vi "Merge Lists.vi"(8 "error in":errorcluster, 9 "new list in":T1[](array[typedef]) {"Last Updated" format="%<%x>T"}, 11 "list in":T1[](array[typedef]) {"Last Updated" format="%<%x>T"}) -> (0 "error out":errorcluster, 3 "list out":T1[](array[typedef]) {"Last Updated" format="%<%x>T"})   [LabVIEW 2018]
uses:
  SR Cluster.ctl
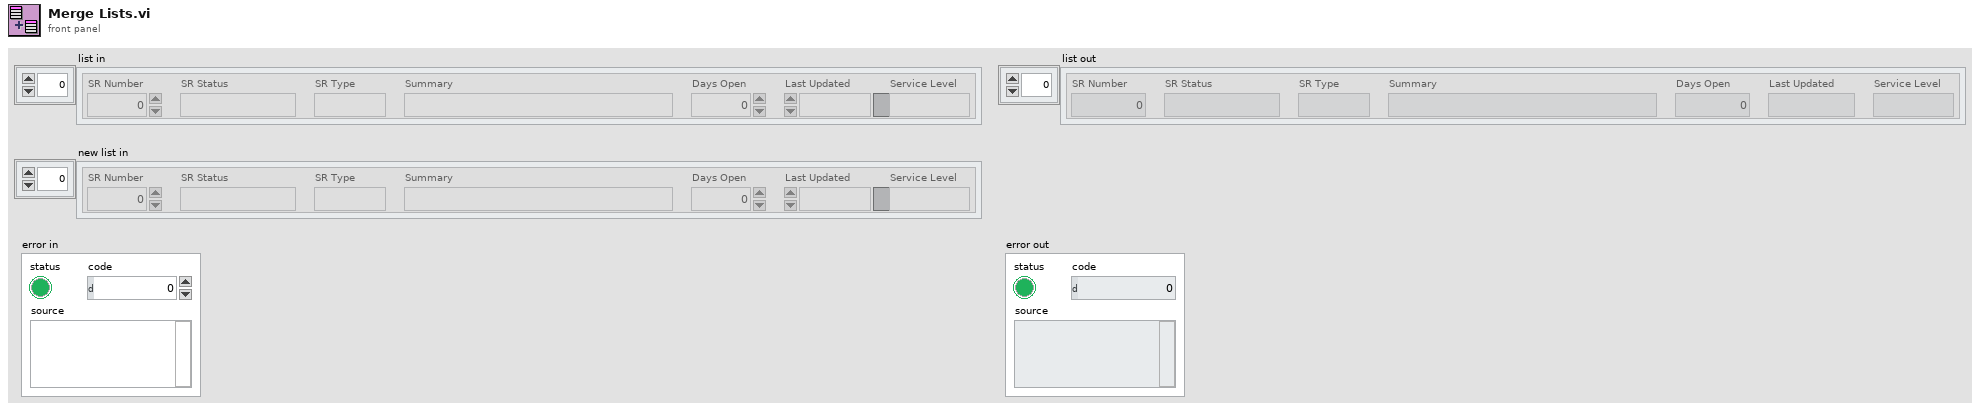
[diagram p1: front panel]
types:
  T1 = typedef "SR Cluster.ctl" = cluster{"SR Number":i32, "SR Status":string, "SR Type":string, "Summary":string, "Days Open":dbl, "Last Updated":timestamp, "Service Level":string}
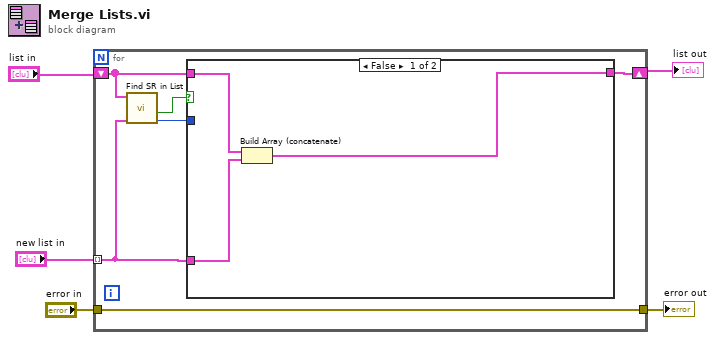
[diagram p0: block diagram]
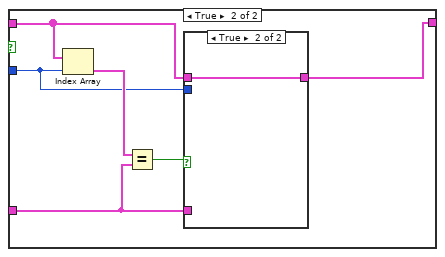
[diagram p2: hidden frame]
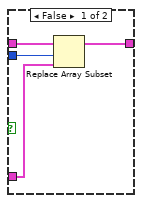
[diagram p3: hidden frame]
diagram:
  n1 = for {
    tunnel: [w11] -> w3
    tunnel: "error in" -> [w11]
    tunnel: "new list in" -> [w8] mode=indexing
    shift-right: [w7] -> w2
    shift-left: "list in" -> [w9]
    n2 = call "Find SR in List.vi"("new SR"=w8, "SR list in"=w9) -> ("SR Index"=w6:i32, "Is SR in List?"=w10:bool)  [unwired: 8 in]
    n3 = case shown="False" w10 {
      tunnel: w9 -> [w14 w18]
      tunnel: w8 -> [w13 w16]
      tunnel: [w12 w15] -> w7
      tunnel: w6 -> [_ w17]
      frame False {
        n4 = Build Array (concatenate)(w14, w13) -> (w12:T1[])
      }
      frame True {
        n5 = Index Array(array=w18, index=w17) -> (element=w19:T1)
        n6 = Equal?(x=w19, y=w16) -> (x = y?=w20:bool)
        n7 = case shown="True" w20 {
          tunnel: w18 -> [w24 w25]
          tunnel: w17 -> [w23 _]
          tunnel: w16 -> [w22 _]
          tunnel: [w21 w25] -> w15
          frame False {
            n8 = Replace Array Subset(array=w24, new element=w22, index=w23) -> (w21:T1[])
          }
          frame True {
          }
        }
      }
    }
  }
  "error out" <- w3
  "list out" <- w2
